vi "ADC contWave cDAQ-9172.vi"(6 "FIN":bool, 9 "Samples":dbl=10000.0, 10 "Sample Rate":dbl=10000.0, 11 "physical channels":tag="cDAQ1Mod1/ai1") -> (0 "error out":errorcluster, 1 "Acquired Data":dbl[](graph), 2 "data":dbl[](array[numeric]) format="%0.2f")   [LabVIEW 2017]
doc: "The DtAinContinuous example demonstrates how to continuously acquire data from an analog input channel. This example runs continuously until either the Stop button is pressed or an error occurs."
uses:
  <vilib>/DAQmx/read.llb/DAQmx Read (Analog 1D DBL 1Chan NSamp).vi
  <vilib>/DAQmx/create/channels.llb/DAQmx Create Channel (AI-Voltage-Basic).vi
  <vilib>/DAQmx/configure/timing.llb/DAQmx Timing (Sample Clock).vi
  <vilib>/DAQmx/miscellaneous.llb/DAQmx Fill In Error Info.vi
panel:
  in  "SampleMode":i32(ring)=10123 items=["Finite Samples"=10178, "Continuous Samples"=10123, "Hardware Timed Single Point"=12522]
  out "Numeric":i32
  # "cDAQ Continuous Analog Input"
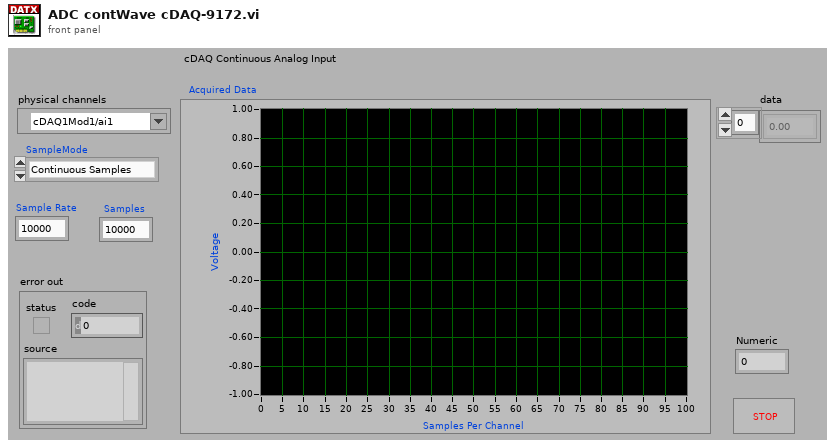
[diagram p1: front panel]
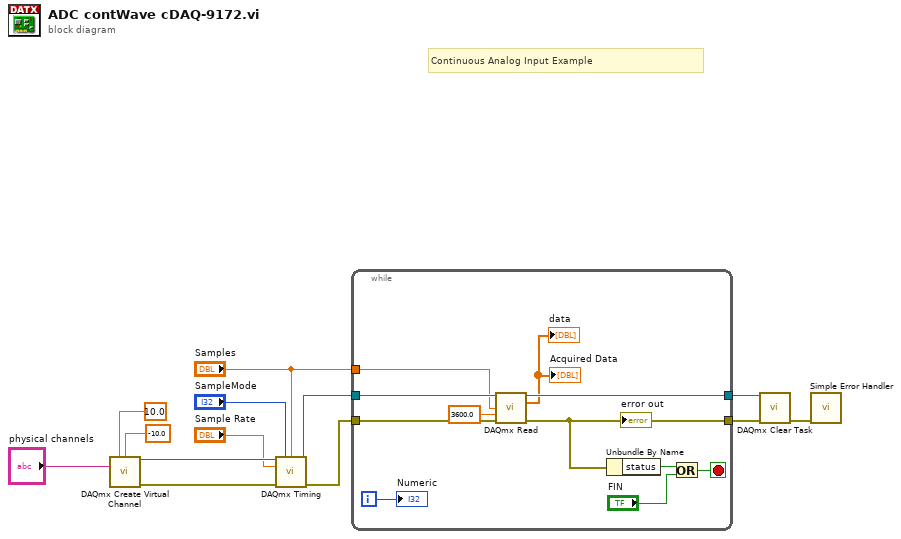
[diagram p0: block diagram]
diagram:
  # "Continuous Analog Input Example"
  n1 = call-poly <vilib>:"DAQmx Create Virtual Channel.vi"("maximum value"=10.0 ("Range Max"), "minimum value"=-10.0 ("Range Min"), "physical channels"="physical channels") -> ("task out"=w7:refnum<k21>, "error out"=w9:errorcluster)  [unwired: 11 in]
  n2 = call-poly <vilib>:"DAQmx Timing.vi"("task/channels in"=w7, "sample mode"="SampleMode", "samples per channel"="Samples", "rate"="Sample Rate", "error in"=w9) -> ("task out"=w6:refnum<k21>, "error out"=w8:errorcluster)  [unwired: 9 in]
  n3 = while {
    tunnel: w8 -> [w22]
    tunnel: [w17] -> w11
    tunnel: w6 -> [w21]
    tunnel: [w20] -> w4
    tunnel: "Samples" -> [w14]
    i -> [w23]
    stop <- w24 stop-if-true
    n4 = call-poly <vilib>:"DAQmx Read.vi"("task/channels in"=w21, "number of samples per channel"=w14, "timeout"=3600.0, "error in"=w22) -> ("task out"=w20:refnum<k21>, "data"=→"Acquired Data" →"data":dbl[], "error out"=w17:errorcluster)  [unwired: 9 in]
    "error out" <- w17
    n5 = Unbundle By Name(w17) -> ("status"=w18:bool)
    n6 = Or(x=w18, y="FIN") -> (x .or. y?=w24:bool)
    "Numeric" <- w23
  }
  n7 = call <vilib>:"DAQmx Clear Task.vi"("task in"=w4, "error in"=w11) -> ("error out"=w10:errorcluster)  [unwired: 13 in]
  n8 = call <vilib>:"Simple Error Handler.vi"("error in (no error)"=w10) -> ()  [unwired: 4 in, 5 out]
